vi "GUI_Frog_HPD.vi"() -> ()   [LabVIEW 2013]
uses:
  Shared/GUI_Template/GUI_master/tcp_new_data_event.ctl
  Shared/GUI_Template/GUI_master/tcp new data cluster.ctl
  GUI_Cameras/Controls/Crosshair type def.ctl
  <vilib>/vision/NI_Vision_Development_Module.lvlib
panel:
  out "Tank":dbl(slide) scale=0.0..255.0 scale format="%#_6p"
  out "131":T1(plugin-control) caption="Spatial Image"
  out "525":T1(plugin-control) caption="FROG Trace"
  out "error out":errorcluster
  in  "Clear":bool
  in  "UDP error message":string
  in  "Refresh Button":bool
  out "GUIdevice 1":string="FrogHPD"
  in  "temporalFWHM::1":dbl caption="Pulse Width" min=0.0 max=50000.0
  in  "Tab Control":T2(tab)
  in  "exposure::1":dbl=0.001 caption="Exposure" min=0.0453 max=10000.0 format="%_4p"
  out "frogerrorfinal::1":dbl caption="Frog Error (<1% OK)" min=0.0 max=500.0
  in  "cameraselect::1":enum16{"temporal CAM", "spatial CAM"}(ring) caption="Select Camera"
  in  "triggermode::1":bool caption="Blank Button"
  out "pulse width":dbl caption="Pulse Width" min=0.0 max=50000.0
  in  "Select device":string(combo)="FrogHPD"
  out "pulse length":cluster{dbl[], dbl[]}(graph)
  out "max counts":cluster{dbl[], dbl[]}(graph)
  out "mean counts":cluster{dbl[], dbl[]}(graph)
  out "Fourier analyzed data":T3
  in  "fourier":bool
  out "SpatialImage::1":T1(plugin-control) caption="Spatial Image"
  out "Time":T4(graph)
  out "Spectrum":T5(graph)
  in  "temporal intensity y::1":dbl[](array[numeric])
  in  "temporal phase y::1":dbl[](array[numeric])
  in  "temporal x::1":dbl[](array[numeric])
  in  "spectrum phase y::1":dbl[](array[numeric])
  in  "spectrum y::1":dbl[](array[numeric])
  in  "spectrum x::1":dbl[](array[numeric])
  out "retrievedFrogTrace::1":T1(plugin-control) caption="Retrieved Frog Trace"
  out "frogTrace::1":T1(plugin-control) caption="FROG Trace"
  in  "insert tag":bool=TRUE
  in  "stop":bool
  out "tcp data event":T6
  out "error IO 2":errorcluster
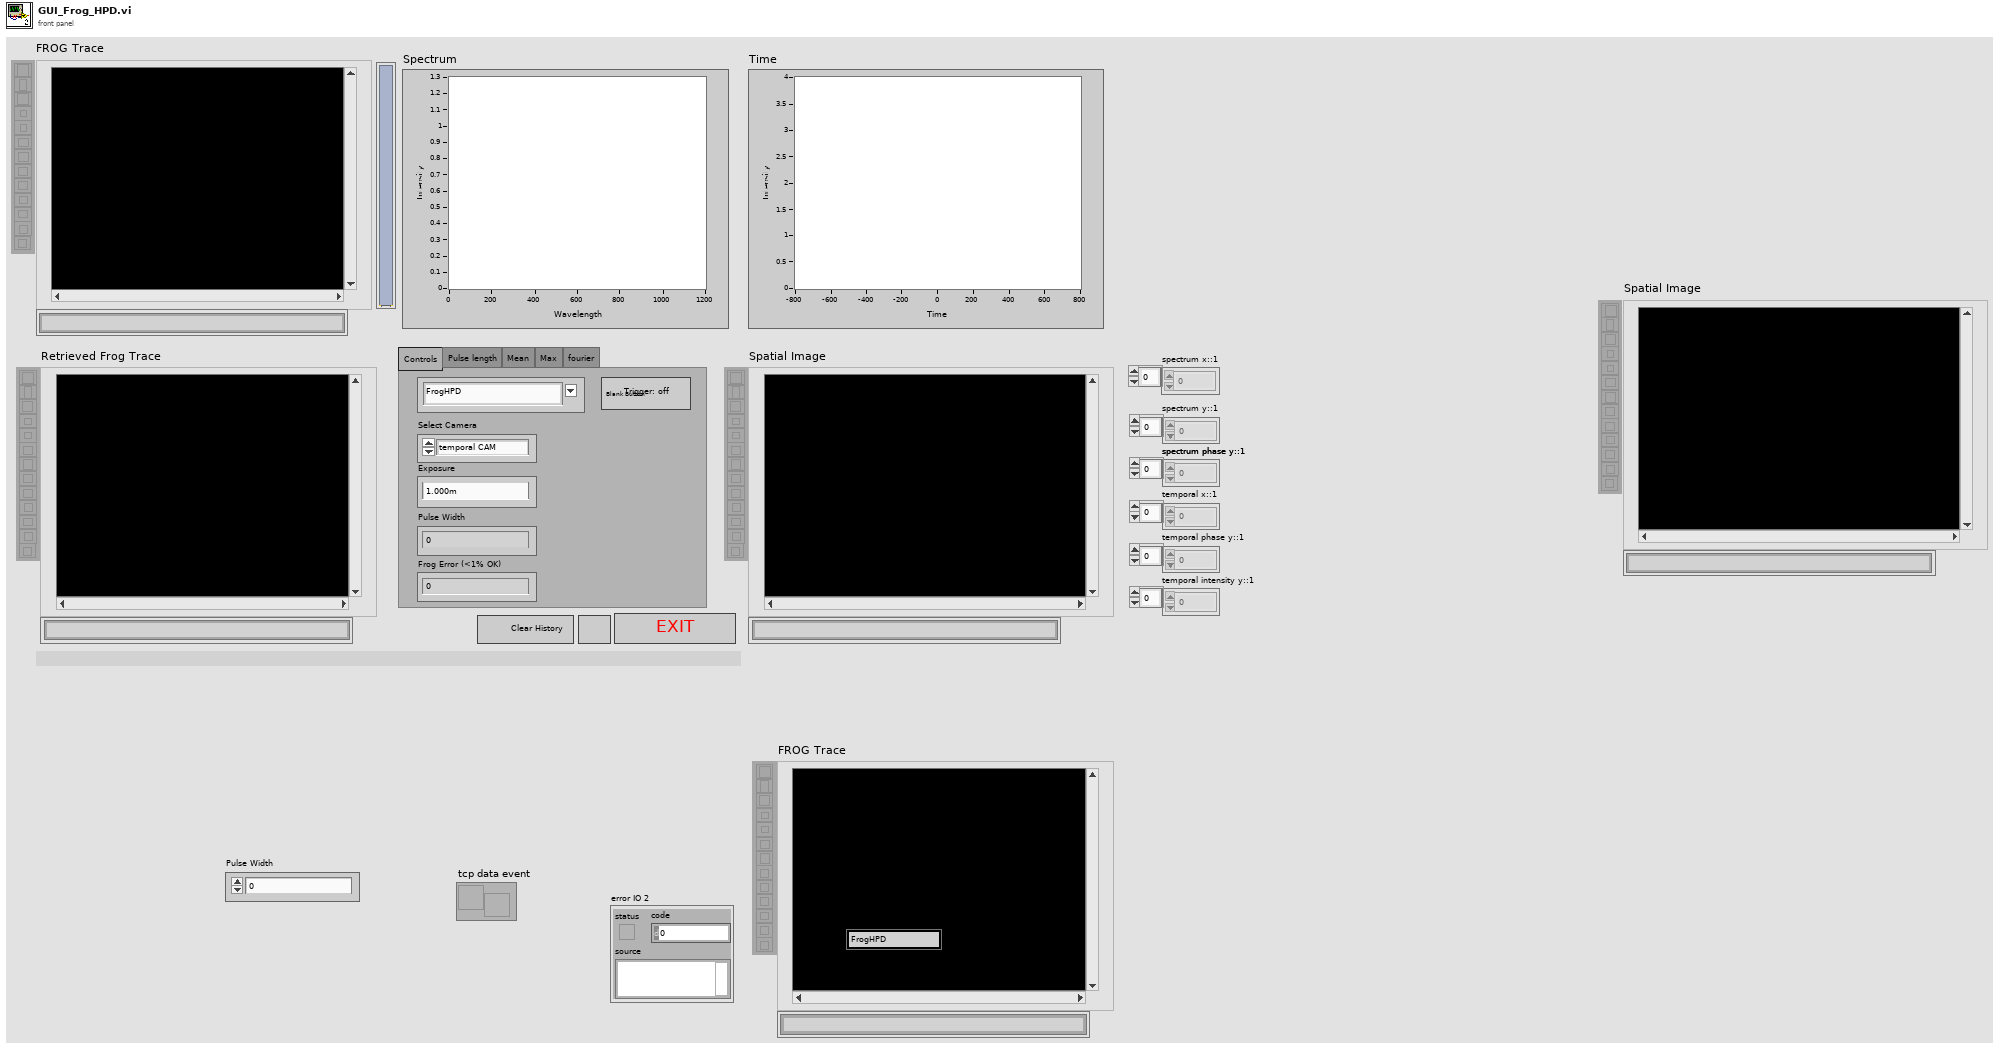
[diagram p1: front panel]
types:
  T1 = typedef "IMAQ Image.ctl" = refnum<image>
  T2 = enum32{"Controls", "Pulse length", "Mean", "Max", "fourier"}
  T3 = cluster{"Amplitude":dbl, "Frequency":dbl, "period":dbl}
  T4 = cluster{"temporal x::1":dbl[], "temporal intensity y::1":dbl[]}[]
  T5 = cluster{"spectrum x::1":dbl[], "spectrum phase y::1":dbl[]}[]
  T6 = typedef "tcp_new_data_event.ctl" = refnum<user-event>
  T7 = typedef "tcp new data cluster.ctl" = cluster{"EventEnum":enum16{"new data", "connection status update"}, "Device name":string}
  T8 = typedef "Crosshair type def.ctl" = cluster{"Draw":bool, "Target":cluster{"x":dbl, "y":dbl}, "Size":cluster{"x":dbl, "y":dbl}, "Angle":dbl, "Color":u32, "Thickness":u8, "CrosshairLabel":string}
  T9 = cluster{"Left":i32, "Top":i32, "Right":i32, "Bottom":i32}
  T10 = typedef "Image Type" = u32
  T11 = cluster{"histogram":u32[], "Minimal Value":sgl, "Maximal Value":sgl, "Starting Value":sgl, "Interval Width":sgl, "Mean Value":sgl, "Standard  Variation":sgl, "Area (pixels)":i32}
  T12 = cluster{"temporal x::1":dbl[], "temporal intensity y::1":dbl[]}
  T13 = cluster{"temporal x::1":dbl[], "temporal phase y::1":dbl[]}
  T14 = cluster{"temporal x::1":dbl[], "temporal phase y::1":dbl[]}[]
  T15 = cluster{"spectrum x::1":dbl[], "spectrum y::1":dbl[]}
  T16 = cluster{"spectrum x::1":dbl[], "spectrum phase y::1":dbl[]}
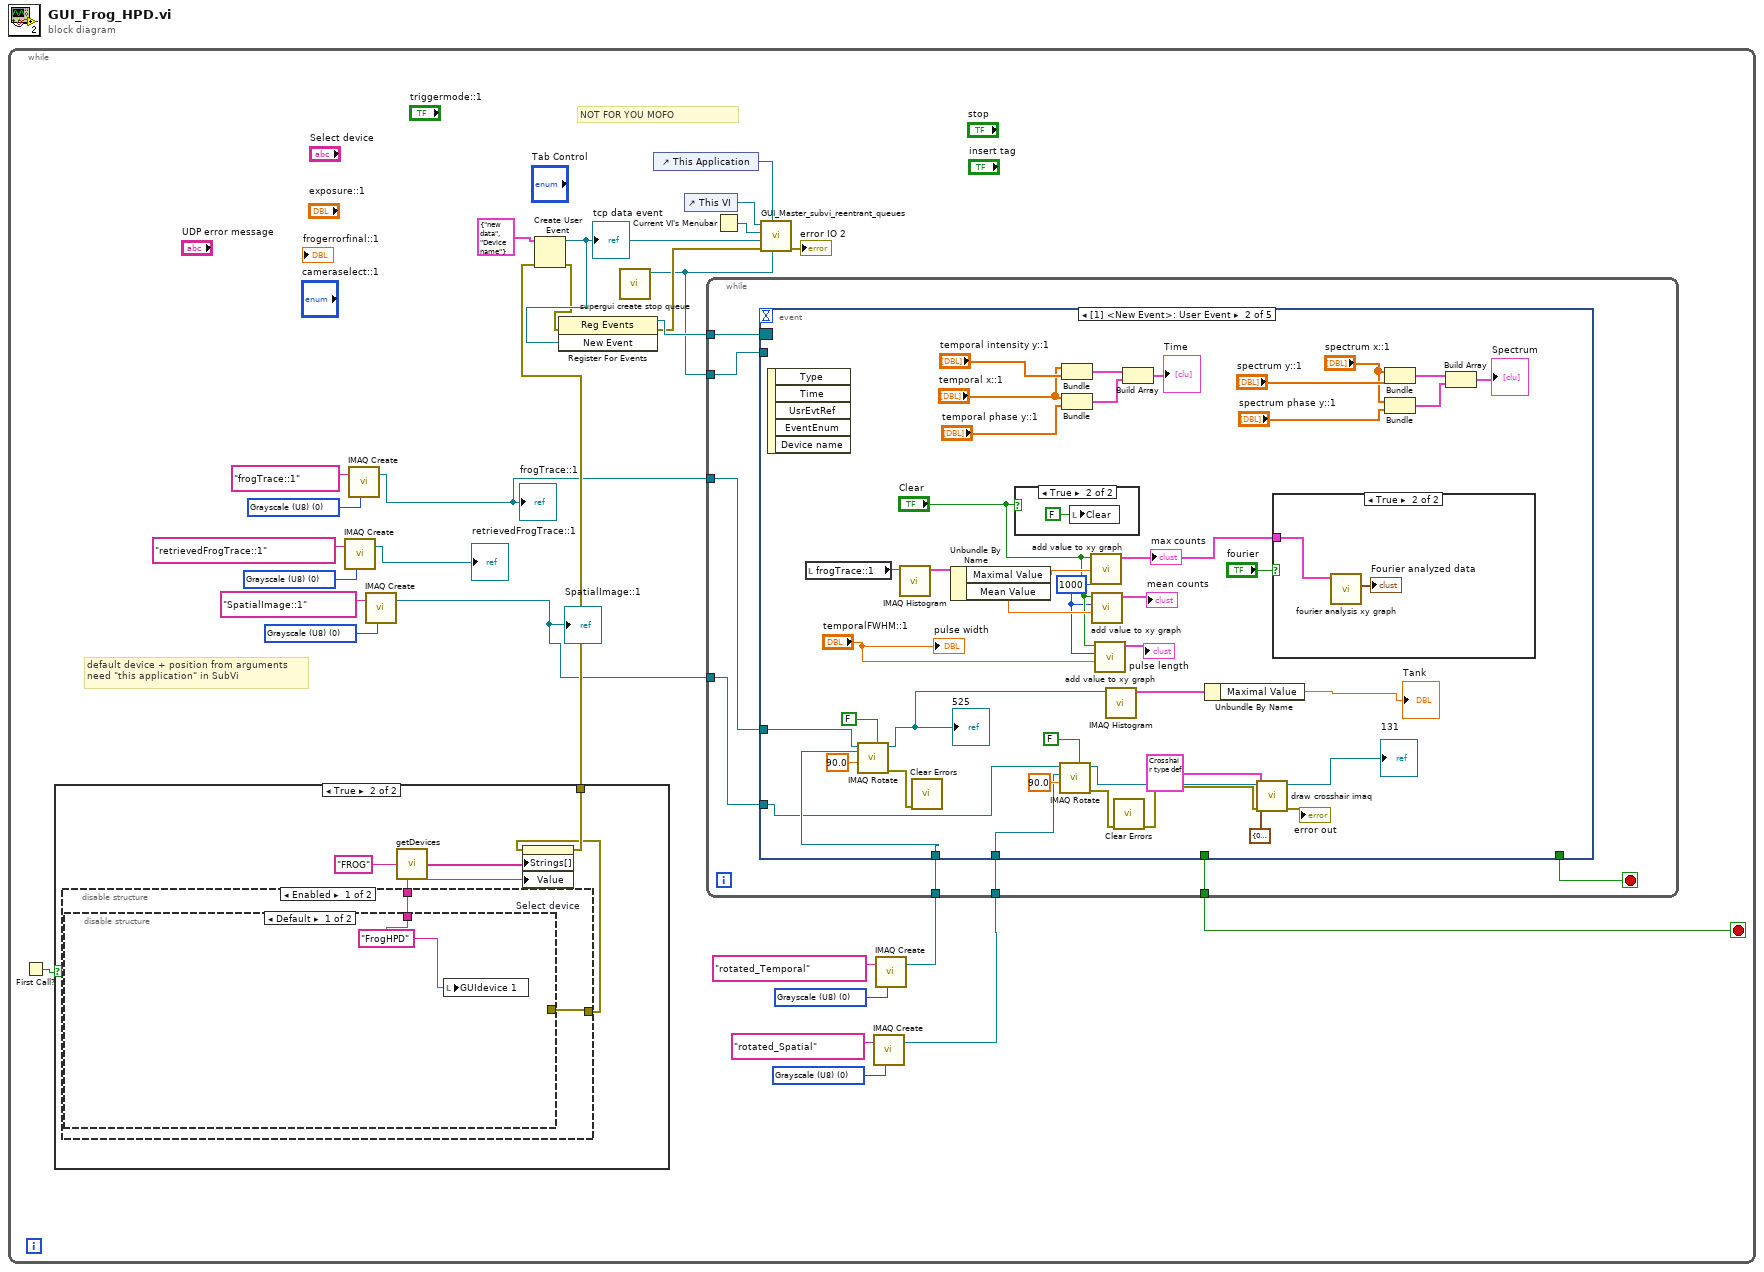
[diagram p0: block diagram]
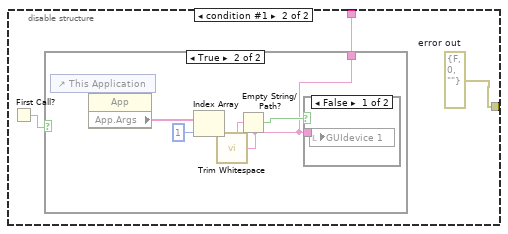
[diagram p3: hidden frame]
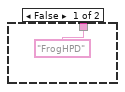
[diagram p4: hidden frame]
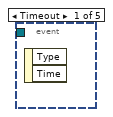
[diagram p7: hidden frame]
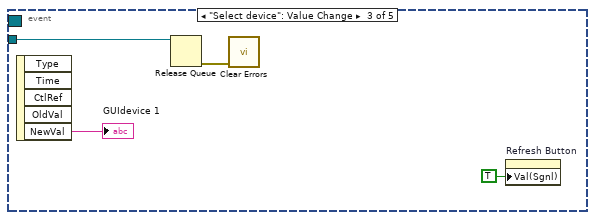
[diagram p10: hidden frame]
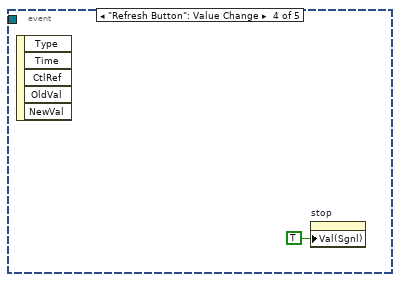
[diagram p11: hidden frame]
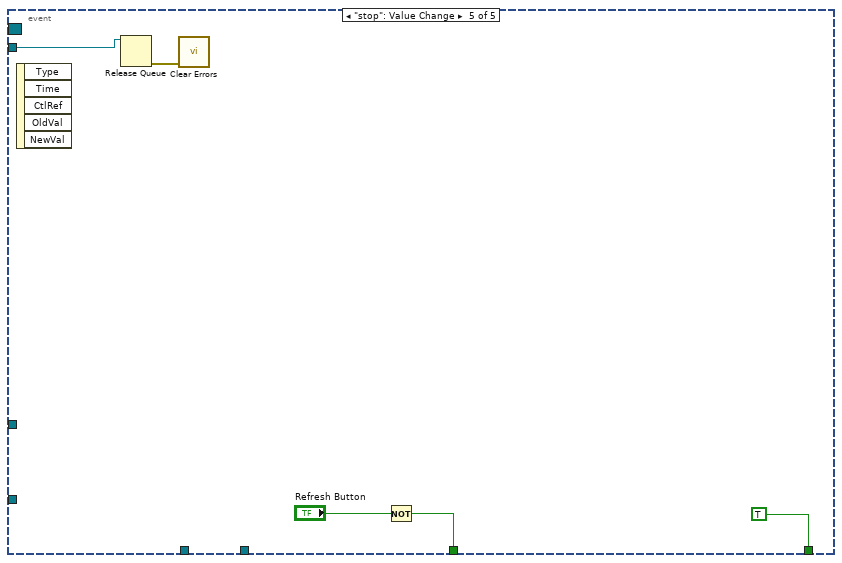
[diagram p12: hidden frame]
diagram:
  n1 = while {
    stop <- w14 stop-if-true
    w4 = T10 0 items=["Grayscale (U8)", "Grayscale (I16)", "Grayscale (SGL)", "Complex (CSG)", "RGB (U32)", "HSL (U32)", "RGB (U64)", "Grayscale (U16)"] ("Image Type")
    w9 = T10 0 items=["Grayscale (U8)", "Grayscale (I16)", "Grayscale (SGL)", "Complex (CSG)", "RGB (U32)", "HSL (U32)", "RGB (U64)", "Grayscale (U16)"] ("Image Type")
    w15 = T10 0 items=["Grayscale (U8)", "Grayscale (I16)", "Grayscale (SGL)", "Complex (CSG)", "RGB (U32)", "HSL (U32)", "RGB (U64)", "Grayscale (U16)"] ("Image Type")
    w19 = T10 0 items=["Grayscale (U8)", "Grayscale (I16)", "Grayscale (SGL)", "Complex (CSG)", "RGB (U32)", "HSL (U32)", "RGB (U64)", "Grayscale (U16)"] ("Image Type")
    w20 = T10 0 items=["Grayscale (U8)", "Grayscale (I16)", "Grayscale (SGL)", "Complex (CSG)", "RGB (U32)", "HSL (U32)", "RGB (U64)", "Grayscale (U16)"] ("Image Type")
    # "default device + position from arguments\nneed \"this application\" in SubVi"
    # "NOT FOR YOU MOFO"
    n2 = First Call?() -> (First Call?: T/F=w10:bool)
    n3 = case shown="True" w10 {
      tunnel: [_ w31] -> w13
      frame False {
      }
      frame True {
        n4 = disable-structure shown="Enabled" {
          disable-tunnel: [w35 _] -> w30
          disable-tunnel: [w34 _] -> w29
          frame Enabled {
            n5 = disable-structure shown="Default" {
              disable-tunnel: [_ w39] -> w35
              disable-tunnel: [w36 w37] -> w34
              frame condition #0 (active) {
                w36 = "FrogHPD" ("trimmed string")
                n6 = local write "GUIdevice 1"(w36) -> ()
              }
              frame condition #1 {
                w39 = errorcluster {"status"=FALSE, "code"=0, "source"=""}  # error out
                n7 = First Call?() -> (First Call?: T/F=w38:bool)
                n8 = case shown="True" w38 {
                  tunnel: ["FrogHPD" ("trimmed string") w41] -> w37
                  frame False {
                  }
                  frame True {
                    n9 = control-ref of="This Application"() -> (w43:refnum<vi>)
                    n10 = property class="App"(reference=w43) -> ("App.Args"=w46:string[])  [unwired: 1 in, 2 out]
                    n11 = Index Array(array=w46, index=1) -> (element=w44:string)
                    n12 = call <vilib>:"Trim Whitespace.vi"("string"=w44) -> ("trimmed string"=w41:string)  [unwired: 1 in]
                    n13 = Empty String/Path?(string/path=w41) -> (empty?=w45:bool)
                    n14 = case shown="False" w45 {
                      tunnel: w41 -> [w47 _]
                      frame False {
                        n15 = local write "GUIdevice 1"(w47) -> ()
                      }
                      frame True {
                      }
                    }
                  }
                }
              }
            }
          }
          frame Disabled {
          }
        }
        n16 = call "getDevices.vi"("Device Class"="FROG") -> ("All Devices"=w32:string[])
        n17 = property on="Select device" class="CmbBox"(error in=w30, "Strings[]"=w32, "Value"=w29) -> (error out=w31:errorcluster)  [unwired: 1 in, 1 out]
      }
    }
    n18 = call "IMAQ Create"("Image Name"="retrievedFrogTrace::1", "Image Type"=w19) -> ("New Image"=→"retrievedFrogTrace::1":T1)  [unwired: 3 in, 1 out]
    n19 = call "IMAQ Create"("Image Name"="frogTrace::1", "Image Type"=w20) -> ("New Image"=w6:T1)  [unwired: 3 in, 1 out]
    "frogTrace::1" <- w6
    n20 = call "IMAQ Create"("Image Name"="SpatialImage::1", "Image Type"=w15) -> ("New Image"=w3:T1)  [unwired: 3 in, 1 out]
    "SpatialImage::1" <- w3
    n21 = Create User Event(user event datatype=T7 {"EventEnum"=enum."new data", "Device name"="Device name"} ("New Event"), error in=w13) -> (user event=w23:refnum<user-event>, error out=w12:errorcluster)
    "tcp data event" <- w23
    n22 = register-events(error in=w12, w23) -> (reference out=w22:refnum<event-registration>, error out=w11:errorcluster)  [unwired: 1 in]
    n23 = call "supergui create stop queue.vi"() -> ("STOP Queue out"=w1:refnum<queue>)  [unwired: 11 in]
    n24 = control-ref of="This Application"() -> (w24:refnum<vi>)
    n25 = control-ref of="This VI"() -> (w27:refnum<vi>)
    n26 = Current VI's Menubar() -> (w26:refnum<k9>)
    n27 = call "GUI_Master_subvi_reentrant_queues.vi"("STOP Queue in"=w1, "This Application"=w24, "error in (no error)"=w11, "tcp data event"=w23, "Caller menu reference"=w26, "Caller VI ref"=w27) -> ("error out"=→"error IO 2":errorcluster)  [unwired: 5 in]
    n28 = call "IMAQ Create"("Image Name"="rotated_Spatial", "Image Type"=w4) -> ("New Image"=w2:T1)  [unwired: 3 in, 1 out]
    n29 = call "IMAQ Create"("Image Name"="rotated_Temporal", "Image Type"=w9) -> ("New Image"=w7:T1)  [unwired: 3 in, 1 out]
    n30 = while {
      tunnel: w22 -> [w54]
      tunnel: [w53] -> w14
      tunnel: w7 -> [w52]
      tunnel: w6 -> [w51]
      tunnel: w3 -> [w50]
      tunnel: w2 -> [w49]
      tunnel: w1 -> [w48]
      stop <- w55 stop-if-true
      n31 = event shown="[1] <New Event>: User Event" {
        selector: w54 -> [_ _ _ _ _]
        dyn-events: _ -> [_ _ _ _ _]
        timeout: _ -> [_ _ _ _ _]
        tunnel: [_ _ _ _ TRUE] -> w55
        tunnel: [_ _ _ _ w108] -> w53
        tunnel: w52 -> [_ w73 _ _ _]
        tunnel: w51 -> [_ w74 _ _ _]
        tunnel: w50 -> [_ w66 _ _ _]
        tunnel: w49 -> [_ w65 _ _ _]
        tunnel: w48 -> [_ _ w102 _ w106]
        event Timeout {
          n32 = event-data() -> ()  [unwired: 1 in, 2 out]
        }
        event User Event {
          w79 = 1000 ("max points")
          n33 = event-data() -> ()  [unwired: 1 in, 5 out]
          n34 = local read "frogTrace::1"() -> (w83:T1)
          n35 = call "IMAQ Rotate"("Maintain Size"=FALSE, "Angle (degrees)"=sgl 90.0, "Image Dst"=w73, "Image Src"=w74) -> ("error out"=w71:errorcluster, "Image Dst Out"=w59:T1)  [unwired: 6 in]
          "525" <- w59
          n36 = call "IMAQ Histogram"("Image"=w83) -> ("Histogram Report"=w85:T11)  [unwired: 9 in, 1 out]
          n37 = call <vilib>:"Clear Errors.vi"("error in (no error)"=w71) -> ()  [unwired: 6 in, 1 out]
          n38 = Unbundle By Name(w85) -> ("Maximal Value"=w84:sgl, "Mean Value"=w82:sgl)
          n39 = case shown="True" "Clear" {
            frame False {
            }
            frame True {
              n40 = local write "Clear"(FALSE ("Clear")) -> ()
            }
          }
          n41 = call "IMAQ Rotate"("Maintain Size"=FALSE, "Angle (degrees)"=sgl 90.0, "Image Dst"=w65, "Image Src"=w66) -> ("error out"=w68:errorcluster, "Image Dst Out"=w62:T1)  [unwired: 6 in]
          n42 = Bundle("temporal x::1"="temporal x::1", "temporal intensity y::1"="temporal intensity y::1") -> (w93:T12)  [unwired: 1 in]
          n43 = Bundle("temporal x::1"="temporal x::1", "temporal phase y::1"="temporal phase y::1") -> (w92:T13)  [unwired: 1 in]
          n44 = call "add value to xy graph.vi"("new value"=w84, "max points"=w79, "Wire in Stop To Clear Graph on Each Run"="Clear") -> ("XY Graph"=w76:cluster{dbl[], dbl[]})  [unwired: 8 in]
          "max counts" <- w76
          n45 = call "add value to xy graph.vi"("new value"=w82, "max points"=w79, "Wire in Stop To Clear Graph on Each Run"="Clear") -> ("XY Graph"=→"mean counts":cluster{dbl[], dbl[]})  [unwired: 8 in]
          n46 = call "add value to xy graph.vi"("new value"="temporalFWHM::1", "max points"=w79, "Wire in Stop To Clear Graph on Each Run"="Clear") -> ("XY Graph"=→"pulse length":cluster{dbl[], dbl[]})  [unwired: 8 in]
          n47 = call "IMAQ Histogram"("Image"=w59) -> ("Histogram Report"=w58:T11)  [unwired: 9 in, 1 out]
          n48 = call <vilib>:"Clear Errors.vi"("error in (no error)"=w68) -> ("error out"=w61:errorcluster)  [unwired: 6 in]
          n49 = Build Array(w93, w92) -> (→"Time":T14)
          n50 = Unbundle By Name(w58) -> ("Maximal Value"=→"Tank":sgl)
          n51 = call "draw crosshair imaq.vi"("error in (no error)"=w61, "Crosshair"=T8 {"Draw"=TRUE, "Target"={"x"=288.0, "y"=384.0}, "Size"={"x"=275.0, "y"=275.0}, "Angle"=0.0, "Color"=14472448, "Thickness"=1, "CrosshairLabel"=""}, "Bounding Rectangle"=T9 {"Left"=0, "Top"=0, "Right"=0, "Bottom"=0}, "image in"=w62) -> ("error out"=→"error out":errorcluster, "image out"=→"131":T1)  [unwired: 6 in]
          n52 = case shown="True" "fourier" {
            tunnel: w76 -> [_ w99]
            frame False {
            }
            frame True {
              n53 = call "fourier analysis xy graph.vi"("xy graph"=w99) -> ("Fourier analyzed data"=→"Fourier analyzed data":T3)  [unwired: 9 in, 1 out]
            }
          }
          n54 = Bundle("spectrum x::1"="spectrum x::1", "spectrum y::1"="spectrum y::1") -> (w86:T15)  [unwired: 1 in]
          n55 = Bundle("spectrum x::1"="spectrum x::1", "spectrum phase y::1"="spectrum phase y::1") -> (w89:T16)  [unwired: 1 in]
          n56 = Build Array(w86, w89) -> (→"Spectrum":T5)
          "pulse width" <- "temporalFWHM::1"
        }
        event "Select device": Value Change {
          n57 = event-data() -> ("NewVal"=→"GUIdevice 1":string)  [unwired: 1 in, 4 out]
          n58 = Release Queue(queue=w102) -> (error out=w101:errorcluster)  [unwired: 2 in, 2 out]
          n59 = call <vilib>:"Clear Errors.vi"("error in (no error)"=w101) -> ()  [unwired: 6 in, 1 out]
          n60 = property on="Refresh Button" class="Bool (strict)"("Val(Sgnl)"=TRUE ("Value (Signaling)")) -> ()  [unwired: 2 in, 2 out]
        }
        event "Refresh Button": Value Change {
          n61 = event-data() -> ()  [unwired: 1 in, 5 out]
          n62 = property on="stop" class="Bool (strict)"("Val(Sgnl)"=TRUE ("Value (Signaling)")) -> ()  [unwired: 2 in, 2 out]
        }
        event "stop": Value Change {
          n63 = event-data() -> ()  [unwired: 1 in, 5 out]
          n64 = Release Queue(queue=w106) -> (error out=w107:errorcluster)  [unwired: 2 in, 2 out]
          n65 = call <vilib>:"Clear Errors.vi"("error in (no error)"=w107) -> ()  [unwired: 6 in, 1 out]
          n66 = Not(x="Refresh Button") -> (.not. x?=w108:bool)
        }
      }
    }
  }
